vi "測定値MAXMIN_G.vi"() -> ()   [LabVIEW 2021]
panel:
  in  "測定値MAX/MINグローバル":string[][](table)
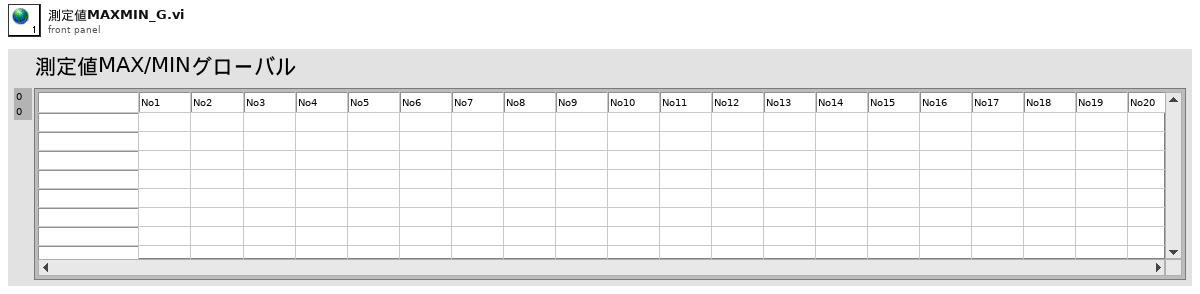
[diagram p1: front panel]
diagram:
